vi "SQL查询.vi"(7 "SQL query":string, 8 "error in (no error)":errorcluster, 11 "database":string) -> (0 "error out":errorcluster, 3 "recordset data":variant[][](array[variant]))   [LabVIEW 2016, in "斯坦道氨氮.lvlib"]
uses:
  <vilib>/Utility/sysdir.llb/System Directory Type.ctl
  <vilib>/addons/database/Connection.llb/DB Tools Open Connec (String).vi
  <vilib>/addons/database/Connection.llb/Conn Execute.vi
  <vilib>/addons/database/Recordset.llb/Rec Fetch Recordset Data (R).vi
  <vilib>/addons/database/Recordset.llb/Rec Destroy - Connection.vi
  <vilib>/addons/database/NI_Database_API.lvlib
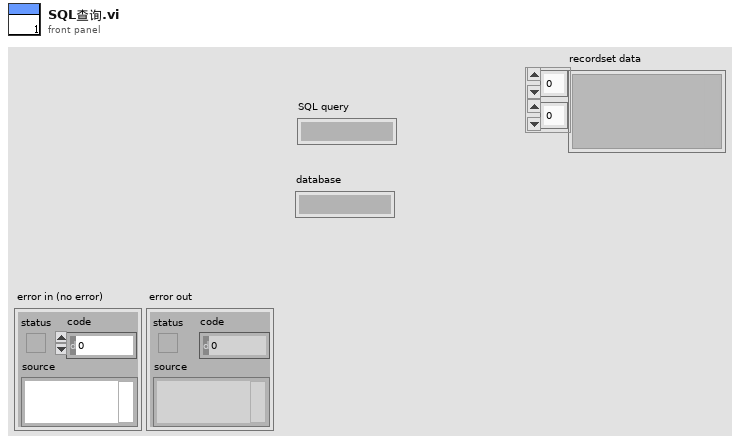
[diagram p1: front panel]
types:
  T1 = typedef "System Directory Type.ctl" = i32
  T2 = typedef "NI_Database_API.lvlib/Conn ObjectReference.ctl" = refnum<k1>
  T3 = typedef "NI_Database_API.lvlib/Rec ObjectReference.ctl" = refnum<k1>
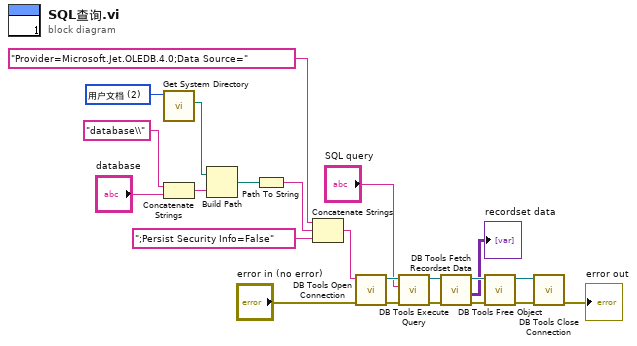
[diagram p0: block diagram]
diagram:
  w20 = T1 2 items=["用户目录"=0, "用户桌面"=1, "用户文档"=2, "用户应用程序数据"=3, "用户设置"=4, "用户临时目录"=5, "公共文档"=6, "公共应用程序数据"=7, "公共设置"=8, "公共缓存"=13, "系统核心库"=9, "系统安装库"=10, "应用程序文件"=11, "启动盘根目录"=12] ("system directory type")
  n1 = call <vilib>:"Get System Directory.vi"("system directory type"=w20) -> ("system directory"=w18:path)  [unwired: 10 in]
  n2 = Concatenate Strings("database\\" ("condition"), "database") -> (w12:string)
  n3 = Build Path(base path=w18, name or relative path=w12) -> (appended path=w17:path)
  n4 = Path To String(path=w17) -> (string=w16:string)
  n5 = Concatenate Strings("Provider=Microsoft.Jet.OLEDB.4.0;Data Source=" ("condition"), w16, ";Persist Security Info=False" ("condition")) -> (w14:string)
  n6 = call-poly <vilib>:"DB Tools Open Connection.vi"("error in (no error)"="error in (no error)", "connection information"=w14) -> ("error out"=w6:errorcluster, "connection reference"=w7:T2)  [unwired: 6 in]
  n7 = call-poly <vilib>:"DB Tools Execute Query.vi"("error in (no error)"=w6, "SQL query"="SQL query", "connection reference"=w7) -> ("error out"=w5:errorcluster, "recordset reference"=w10:T3)  [unwired: 5 in]
  n8 = call-poly <vilib>:"DB Tools Fetch Recordset Data.vi"("error in (no error)"=w5, "recordset reference"=w10) -> ("error out"=w8:errorcluster, "recordset data"=→"recordset data":variant[][], "recordset reference out"=w9:T3)  [unwired: 3 in]
  n9 = call-poly <vilib>:"DB Tools Free Object.vi"("error in (no error)"=w8, "recordset reference"=w9) -> ("error out"=w3:errorcluster, "connection reference"=w4:T2)  [unwired: 8 in]
  n10 = call <vilib>:"DB Tools Close Connection.vi"("error in (no error)"=w3, "connection reference"=w4) -> ("error out"=→"error out":errorcluster)  [unwired: 5 in]
